vi "Logging Message Loop.vi"(8 "error in (no error)":errorcluster, 10 "Data Queue":refnum<queue>, 11 "Message Queues":T1) -> (0 "error out":errorcluster)   [LabVIEW 2013, in "Logging.lvlib"]
doc: "The message loop subVI to handle messages pertaining to logging data."
uses:
  Logging.lvlib
  support/Message Queue/All Message Queues.ctl
  support/Message Queue/Message Cluster.ctl
  Logging Configuration.ctl
  Logging State.ctl
  controls/UI Data.ctl
  <vilib>/Utility/error.llb/DialogType.ctl
  support/Message Queue/Enqueue Message (Single).vi
  <vilib>/ErrorRing/Error Ring.xnode
  support/Message Queue/Message Queue.lvlib
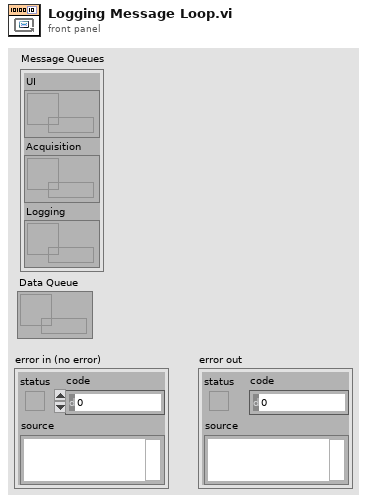
[diagram p1: front panel]
types:
  T1 = typedef "Message Queue.lvlib/All Message Queues.ctl" = cluster{"UI":refnum<queue>, "Acquisition":refnum<queue>, "Logging":refnum<queue>}
  T2 = cluster{"Macro:Initialize":string, "Macro:Exit":string, "Core":cluster{"Current VI Reference":refnum<vi>, "Close Panel on Exit?":bool}}
  T3 = typedef "UI Data.ctl" = cluster{"Start Ref":refnum<vi>, "Stop Ref":refnum<vi>, "Settings Ref":refnum<vi>, "Exit Ref":refnum<vi>, "Status Ref":refnum<vi>, "Data Ref":refnum<vi>}
  T4 = typedef "Logging.lvlib/Logging State.ctl" = enum16{"Idle", "Logging"}
  T5 = typedef "Logging.lvlib/Logging Configuration.ctl" = cluster{"Log File Base Path":path, "TDMS File Reference":refnum<k34>}
  T6 = enum32{"invalid app kind", "Development System", "Run Time System", "Student Edition", "Embedded LabVIEW", "Evaluation", "Custom"}
  T7 = typedef "Message Queue.lvlib/Message Cluster.ctl" = cluster{"Message":string, "Message Data":variant}
  T8 = enum32{"Invalid", "Standard", "Closed", "Hidden", "Minimized", "Maximized"}
  T9 = enum16{"open", "open or create", "create or replace", "create", "open (read-only)"}
  T10 = typedef "DialogType.ctl" = u16
  T11 = cluster{"element":T7, "error constant":errorcluster}
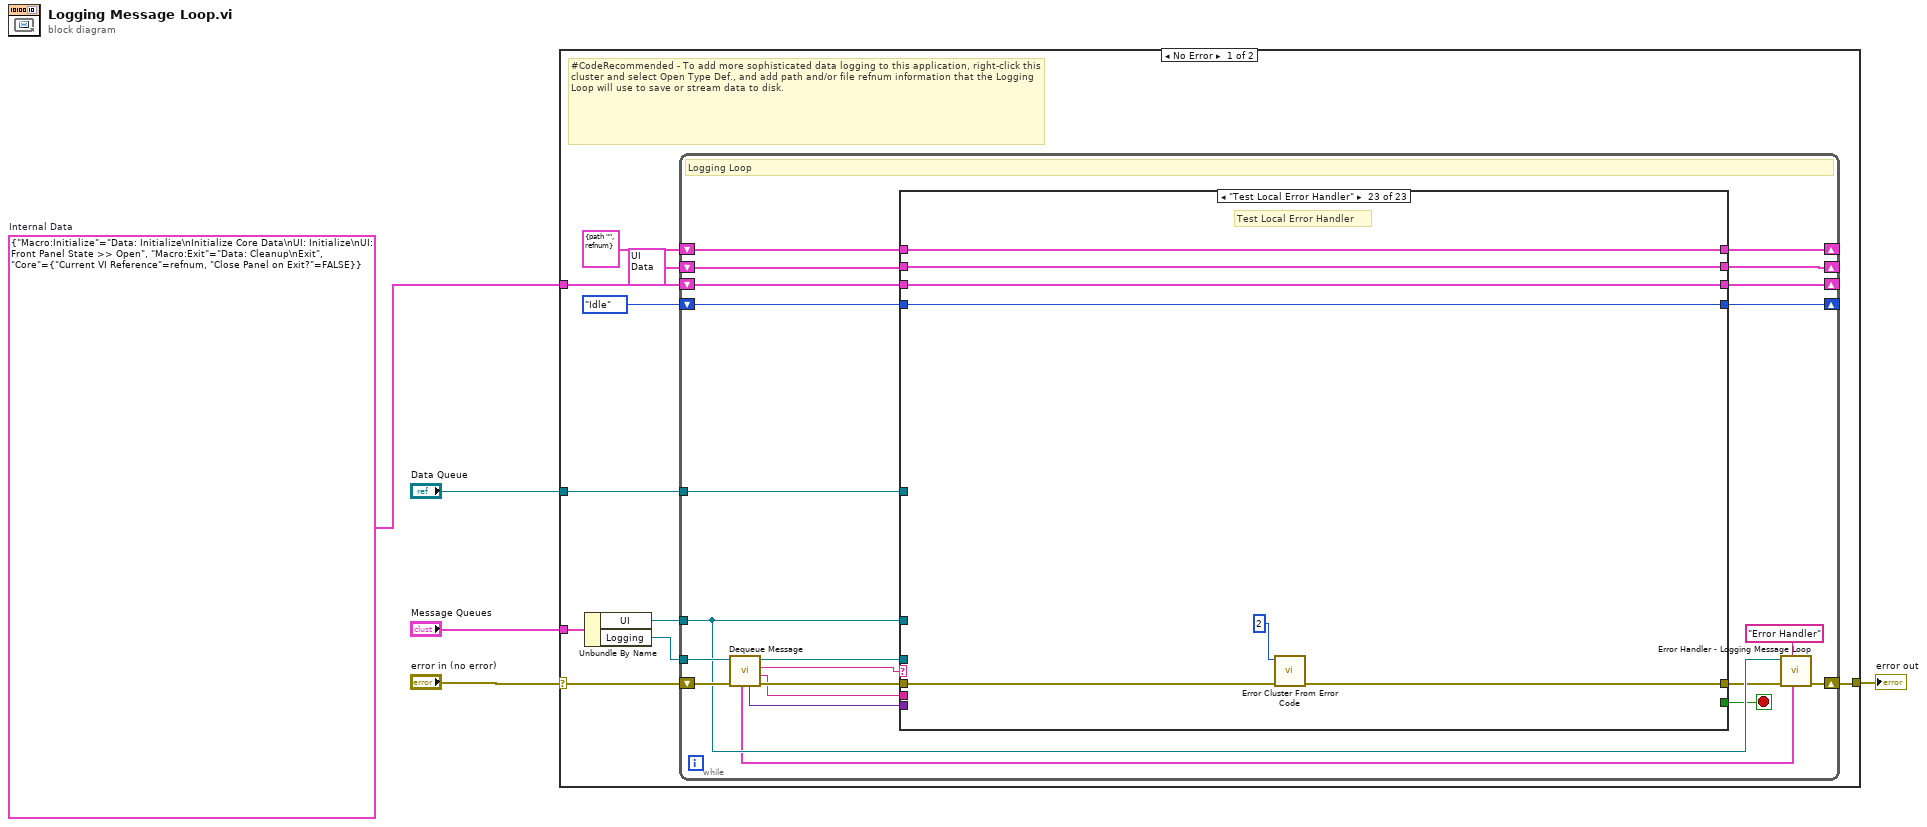
[diagram p0: block diagram]
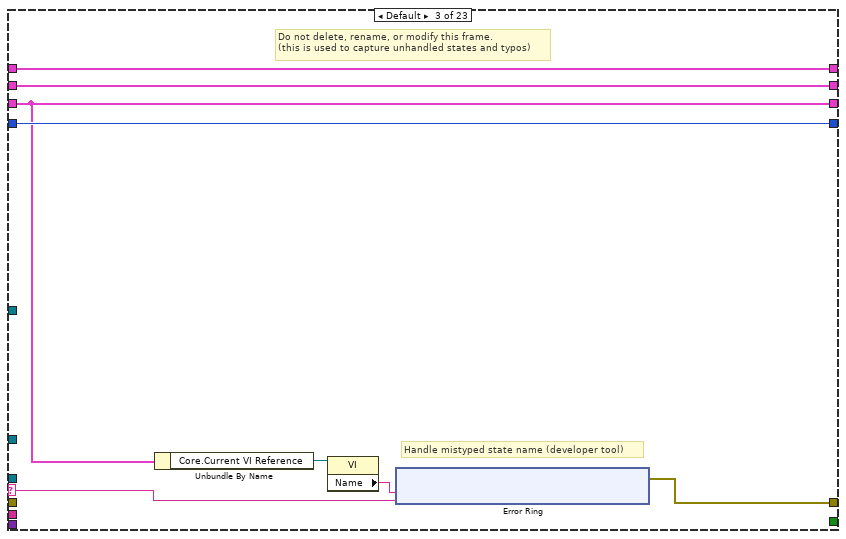
[diagram p4: hidden frame]
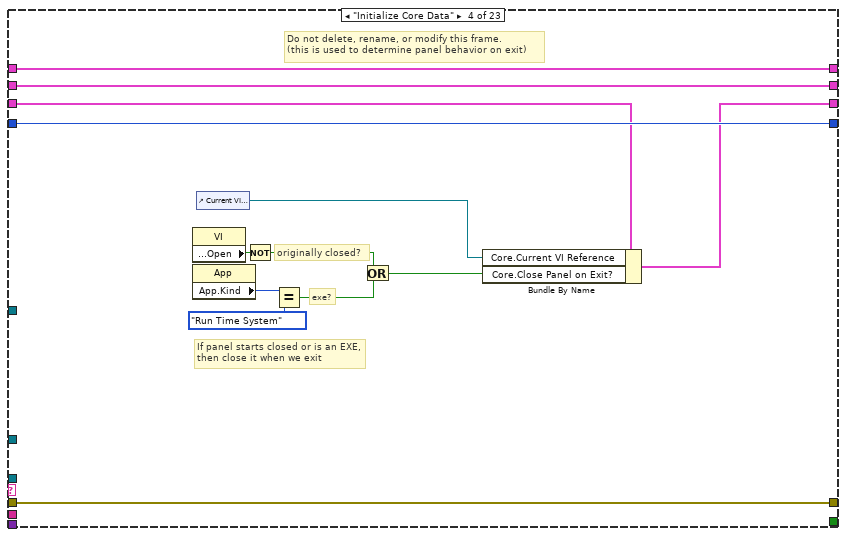
[diagram p5: hidden frame]
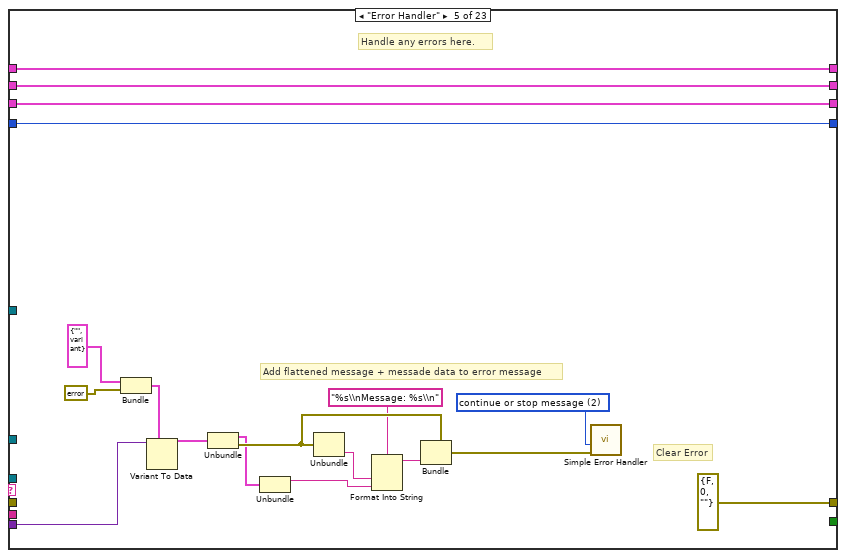
[diagram p6: hidden frame]
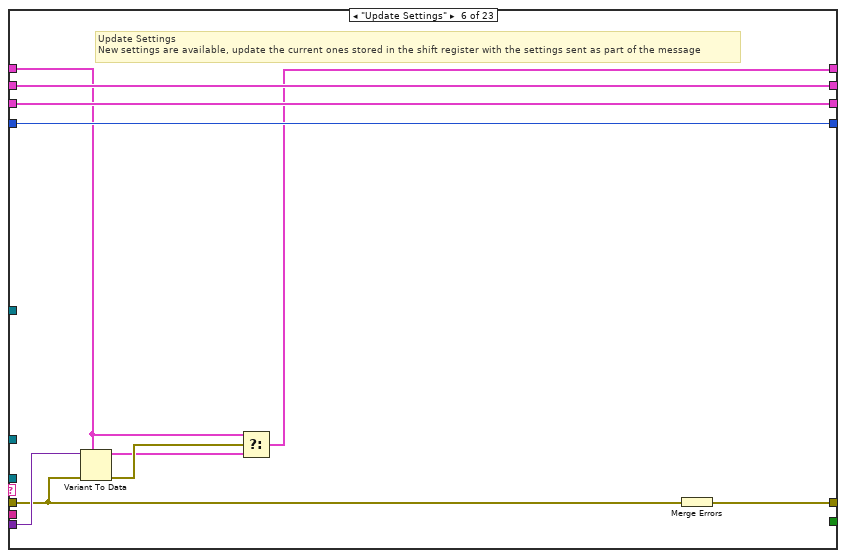
[diagram p7: hidden frame]
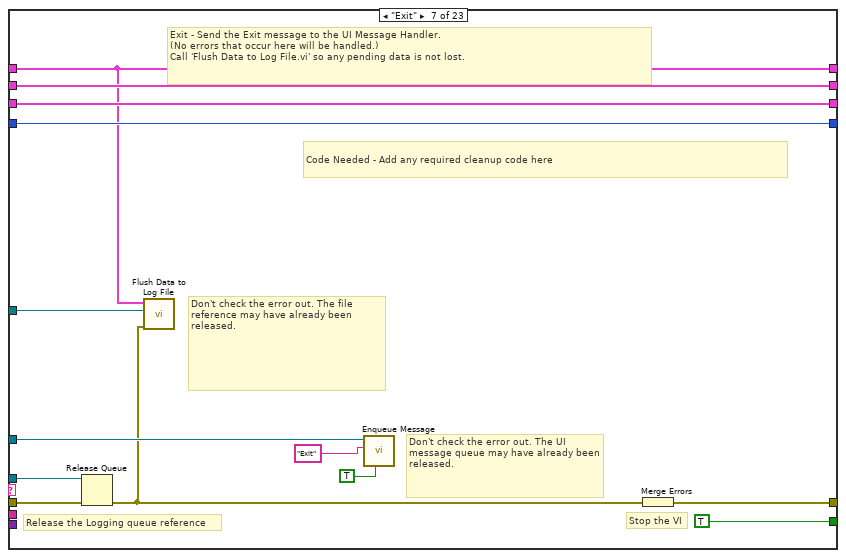
[diagram p8: hidden frame]
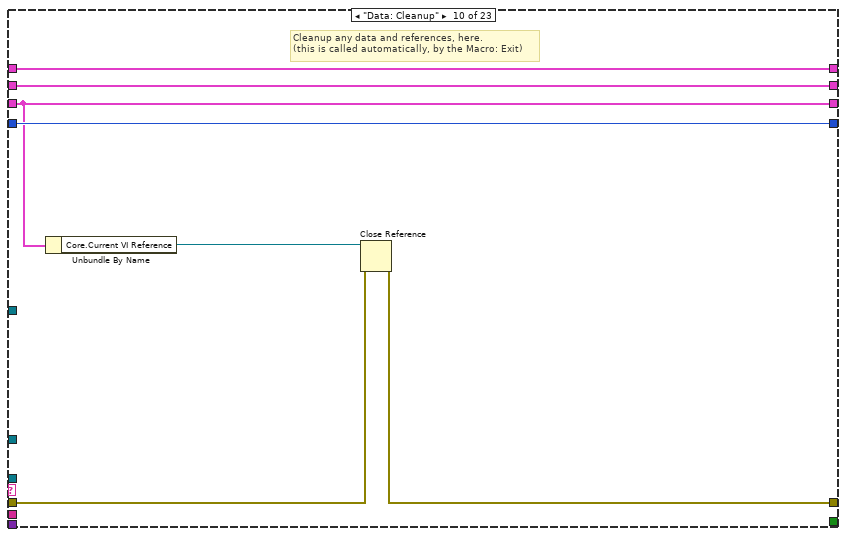
[diagram p11: hidden frame]
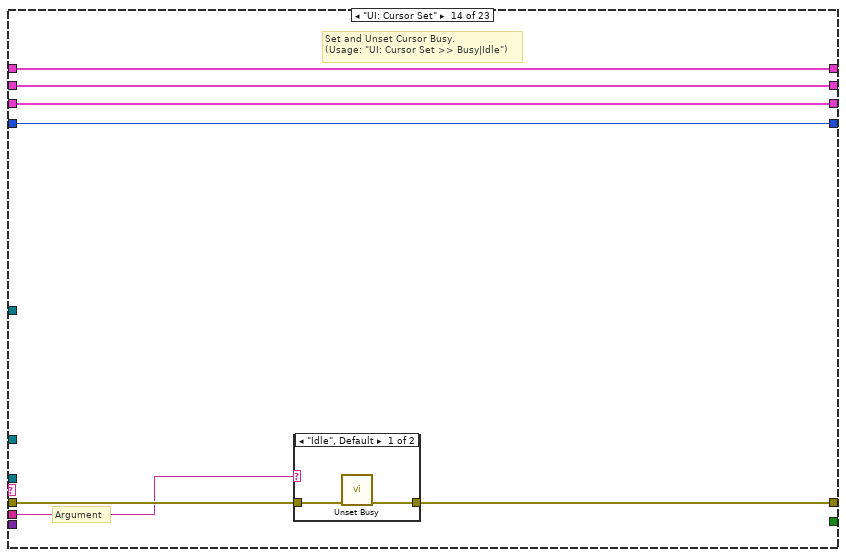
[diagram p15: hidden frame]
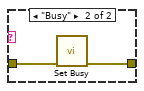
[diagram p16: hidden frame]
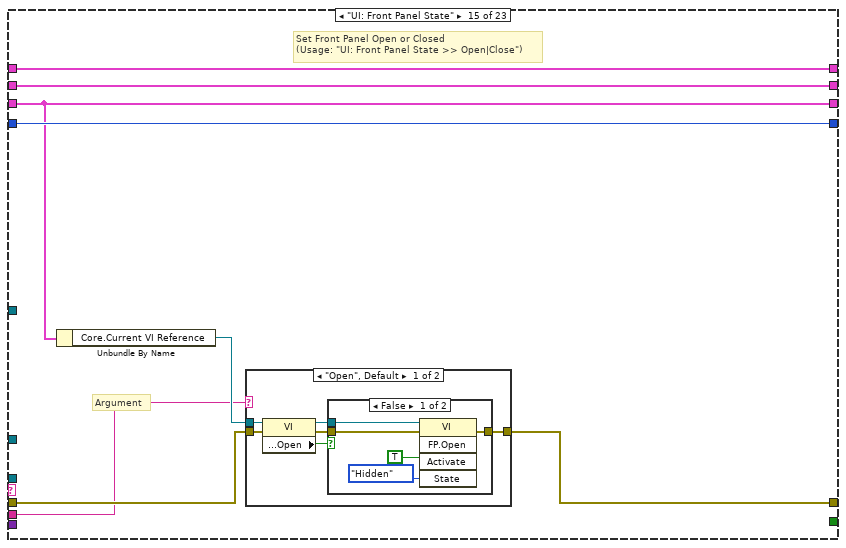
[diagram p17: hidden frame]
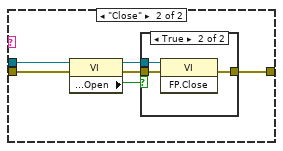
[diagram p19: hidden frame]
diagram:
  w1 = T2 {"Macro:Initialize"="Data: Initialize\nInitialize Core Data\nUI: Initialize\nUI: Front Panel State >> Open", "Macro:Exit"="Data: Cleanup\nExit", "Core"={"Current VI Reference"=refnum, "Close Panel on Exit?"=FALSE}}  # Internal Data
  n1 = case shown="No Error" "error in (no error)" {
    selector: "error in (no error)" -> [w11 w307]
    tunnel: "Message Queues" -> [w15 _]
    tunnel: [w13 w307] -> w4
    tunnel: "Data Queue" -> [w10 _]
    tunnel: w1 -> [w7 _]
    frame No Error {
      # "#CodeRecommended - To add more sophisticated data logging to this application, right-click this cluster and select Open Type Def., and add path and/or file refnum information that the Logging Loop will use to save or stream data to disk."
      n2 = Unbundle By Name(w15) -> ("UI"=w9:refnum<queue>, "Logging"=w14:refnum<queue>)
      n3 = while {
        tunnel: w14 -> [w36]
        shift-right: [w25] -> _
        shift-left: T5 {"Log File Base Path"=path "", "TDMS File Reference"=refnum} ("Logging Configuration") -> [w26]
        shift-right: [w35] -> w13
        shift-left: w11 -> [w37]
        tunnel: w9 -> [w33]
        tunnel: w10 -> [w20]
        shift-right: [w23] -> _
        shift-left: Logging_State."Idle" ("State") -> [w24]
        shift-right: [w19] -> _
        shift-left: T3 {"Start Ref"=refnum, "Stop Ref"=refnum, "Settings Ref"=refnum, "Exit Ref"=refnum, "Status Ref"=refnum, "Data Ref"=refnum} ("Measurement UI Controls") -> [w21]
        shift-right: [w18] -> _
        shift-left: w7 -> [w22]
        stop <- w28 stop-if-true
        # "Logging Loop"
        n4 = call "Dequeue Message.vi"("error in (no error)"=w37, "Message Queue"=w36) -> ("error out"=w34:errorcluster, "Argument"=w30:string, "Message"=w31:string, "dup Message Queue"=w32:refnum<queue>, "Message Data"=w29:variant, "element"=w16:T7)  [unwired: 4 in]
        n5 = case shown="\"Test Local Error Handler\"" w31 {
          selector: w31 -> [_ _ w50 _ _ _ _ _ _ _ _ _ _ _ _ _ _ _ _ _ w261 _ _]
          tunnel: w21 -> [w41 w45 w54 w68 w94 w104 w116 w120 w127 w130 w137 w142 w147 w152 w163 w193 w202 w216 w222 w229 w264 w288 w305]
          tunnel: w30 -> [_ _ _ _ _ _ _ _ _ _ _ _ _ w153 w164 _ _ _ _ _ _ _ _]
          tunnel: w26 -> [w40 w46 w55 w66 w92 w98 w106 w121 w123 w131 w138 w144 w149 w156 w166 w194 w203 w214 w223 w230 w259 w279 w304]
          tunnel: [w42 w47 w48 w76 errorcluster {"status"=FALSE, "code"=0, "source"=""} ("error out") w96 w108 w122 w124 w132 w139 w143 w148 w154 w167 w195 w198 w204 w224 w227 w262 w284 w300] -> w27
          tunnel: w34 -> [w42 w47 _ w76 _ w95 w113 w122 w124 w133 w139 w143 w148 w155 w168 w195 w200 w213 w224 w226 w260 w283 w301]
          tunnel: [w41 w45 w54 w68 w94 w104 w116 w120 w127 w130 w137 w142 w147 w152 w163 w193 w202 w216 w222 w229 w264 w288 w305] -> w19
          tunnel: [_ _ _ _ _ _ TRUE _ _ _ _ _ _ _ _ _ _ _ _ _ _ _ _] -> w28
          tunnel: [w40 w46 w55 w66 w92 w97 w106 w121 w123 w131 w138 w144 w149 w156 w166 w194 w203 w214 w223 w231 w259 w278 w304] -> w25
          tunnel: [w39 w44 w53 w67 w93 w103 w115 w119 w126 w129 w136 w141 w146 w151 w162 w192 w201 w215 w221 w228 w263 w286 w303] -> w23
          tunnel: w24 -> [w39 w44 w53 w67 w93 w103 w115 w119 w126 w129 w136 w141 w146 w151 w162 w192 w201 w215 w221 w232 w265 w287 w303]
          tunnel: w29 -> [_ _ _ _ w77 w101 _ _ _ _ _ _ _ _ _ _ _ _ _ _ _ _ _]
          tunnel: w22 -> [w38 w43 w49 w65 w91 w102 w114 w118 w125 w128 w135 w140 w145 w150 w161 w191 w196 w207 w220 w233 w266 w289 w306]
          tunnel: [w38 w43 w49 w64 w91 w102 w114 w118 w125 w128 w135 w140 w145 w150 w161 w191 w196 w207 w220 w233 w266 w289 w306] -> w18
          tunnel: w32 -> [_ _ _ _ _ _ w112 _ _ _ _ _ _ _ _ _ w199 w212 _ w225 w257 _ _]
          tunnel: w33 -> [_ _ _ _ _ _ w111 _ _ _ _ _ _ _ _ _ _ _ _ _ _ w281 _]
          tunnel: w20 -> [_ _ _ _ _ _ w107 _ _ _ _ _ _ _ _ _ _ _ _ _ w258 w282 _]
          frame "", "Idle" {
            # "Executes when the state queue is empty\nAlso commented out messages"
          }
          frame "---------- Core ----------" {
            # "Do not put any code in this frame.\n(it is a separator no-op)"
          }
          frame Default {
            # "Handle mistyped state name (developer tool)"
            # "Do not delete, rename, or modify this frame.\n(this is used to capture unhandled states and typos)"
            n6 = Unbundle By Name(w49) -> ("Core.Current VI Reference"=w51:refnum<vi>)
            n7 = property class="VI"(reference=w51) -> ("Name"=w52:string)  [unwired: 1 in, 2 out]
            n8 = xnode "Error Ring"("parameter 0"=w52, "parameter 1"=w50) -> ("error out"=w48:errorcluster)
          }
          frame "Initialize Core Data" {
            # "Do not delete, rename, or modify this frame.\n(this is used to determine panel behavior on exit)"
            # "originally closed?"
            # "exe?"
            # "If panel starts closed or is an EXE, then close it when we exit"
            n9 = property class="VI"() -> ("Front Panel.Open"=w75:bool)  [unwired: 2 in, 2 out]
            n10 = property class="App"() -> ("App.Kind"=w74:T6)  [unwired: 2 in, 2 out]
            n11 = control-ref of="Current VI Reference"() -> (w69:refnum<vi>)
            n12 = Not(x=w75) -> (.not. x?=w72:bool)
            n13 = Equal?(x=w74, y=T6."Run Time System" ("Application:Kind")) -> (x = y?=w71:bool)
            n14 = Or(x=w72, y=w71) -> (x .or. y?=w70:bool)
            n15 = Bundle By Name(cluster=w65, "Core.Current VI Reference"=w69, "Core.Close Panel on Exit?"=w70) -> (w64:T2)
          }
          frame "Error Handler" {
            w89 = T10 2 items=["no dialog", "OK message", "continue or stop message", "OK message + warnings", "continue/stop + warnings"] ("type of dialog (OK msg:1)")
            # "Add flattened message + messade data to error message"
            # "Clear Error"
            # "Handle any errors here."
            n16 = Bundle("element"=T7 {"Message"="", "Message Data"=variant}, "error constant"=errorcluster {"status"=FALSE, "code"=0, "source"=""}) -> (w86:T11)  [unwired: 1 in]
            n17 = Variant To Data(type=w86, Variant=w77) -> (data=w85:T11)  [unwired: 1 in, 1 out]
            n18 = Unbundle(w85) -> ("element"=w82:T7, "error constant"=w84:errorcluster)
            n19 = Unbundle(w82) -> ("Message"=w80:string)  [unwired: 1 out]
            n20 = Unbundle(w84) -> ("source"=w79:string)  [unwired: 2 out]
            n21 = Format Into String(format string="%s\\nMessage: %s\\n", w79, w80) -> (resulting string=w81:string)  [unwired: 2 in, 1 out]
            n22 = Bundle(cluster=w84, "source"=w81) -> (w83:errorcluster)  [unwired: 2 in]
            n23 = call <vilib>:"Simple Error Handler.vi"("type of dialog (OK msg:1)"=w89, "error in (no error)"=w83) -> ()  [unwired: 3 in, 5 out]
          }
          frame "Update Settings" {
            # "Update Settings\nNew settings are available, update the current ones stored in the shift register with the settings sent as part of the message"
            n24 = Variant To Data(error in=w95, type=w98, Variant=w101) -> (data=w99:T5, error out=w100:errorcluster)
            n25 = Select(t=w98, s=w100, f=w99) -> (s? t:f=w97:T5)
            n26 = Merge Errors(w95) -> (w96:errorcluster)
          }
          frame "Exit" {
            # "Stop the VI"
            # "Don't check the error out. The file reference may have already been released."
            # "Code Needed - Add any required cleanup code here"
            # "Exit - Send the Exit message to the UI Message Handler.\n(No errors that occur here will be handled.)\nCall 'Flush Data to Log File.vi' so any pending data is not lost."
            # "Don't check the error out. The UI message queue may have already been released."
            # "Release the Logging queue reference"
            n27 = Release Queue(queue=w112, error in (no error)=w113) -> (error out=w105:errorcluster)  [unwired: 1 in, 2 out]
            n28 = call "Flush Data to Log File.vi"("error in (no error)"=w105, "Data Queue"=w107, "Logging Configuration"=w106) -> ()  [unwired: 8 in, 1 out]
            n29 = call-poly "Enqueue Message.vi"("Priority Message? (F)"=TRUE, "Message"="Exit", "Message Queue"=w111) -> ()  [unwired: 7 in, 2 out]
            n30 = Merge Errors(w105) -> (w108:errorcluster)
          }
          frame "---------- Data ----------" {
            # "Do not put any code in this frame.\n(It is a separator no-op. You can make a copy of this frame to create a new Data frame)"
          }
          frame "Data: Initialize" {
            # "nothing right now"
            # "Initialize the shift-register data, here.\n(data names are defined by what you wire into the bundle function)"
          }
          frame "Data: Cleanup" {
            # "Cleanup any data and references, here.\n(this is called automatically, by the Macro: Exit)"
            n31 = Unbundle By Name(w128) -> ("Core.Current VI Reference"=w134:refnum<vi>)
            n32 = Close Reference(reference=w134, error in (no error)=w133) -> (error out=w132:errorcluster)
          }
          frame "---------- UI ----------" {
            # "Do not put any code in this frame.\n(It is a separator no-op. You can make a copy of this frame to create a new UI frame)"
          }
          frame "UI: Initialize" {
            # "Initialize the User Interface, here.\n(this is called automatically, by the Macro: Init)"
          }
          frame "UI: Initialize UI Refs" {
            # "Package and Init UI Refs as Required"
          }
          frame "UI: Cursor Set" {
            # "Argument"
            # "Set and Unset Cursor Busy.\n(Usage: \"UI: Cursor Set >> Busy|Idle\")"
            n33 = case shown="\"Idle\", Default" w153 {
              tunnel: w155 -> [w158 w160]
              tunnel: [w157 w159] -> w154
              frame "Idle", Default {
                n34 = call <vilib>:"Unset Busy.vi"("error in (no error)"=w158) -> ("error out"=w157:errorcluster)  [unwired: 10 in]
              }
              frame "Busy" {
                n35 = call <vilib>:"Set Busy.vi"("error in (no error)"=w160) -> ("error out"=w159:errorcluster)  [unwired: 9 in, 1 out]
              }
            }
          }
          frame "UI: Front Panel State" {
            # "Argument"
            # "Set Front Panel Open or Closed\n(Usage: \"UI: Front Panel State >> Open|Close\")"
            n36 = Unbundle By Name(w161) -> ("Core.Current VI Reference"=w165:refnum<vi>)
            n37 = case shown="\"Open\", Default" w164 {
              tunnel: w168 -> [w172 w185]
              tunnel: [w174 w186] -> w167
              tunnel: w165 -> [w173 w183]
              frame "Open", Default {
                n38 = property class="VI"(reference=w173, error in=w172) -> (reference out=w170:refnum<vi>, error out=w171:errorcluster, "Front Panel.Open"=w169:bool)
                n39 = case shown="False" w169 {
                  tunnel: [w177 w180] -> w174
                  tunnel: w171 -> [w176 w180]
                  tunnel: w170 -> [w175 _]
                  frame False {
                    n40 = invoke class="VI" method="FP.Open"(reference=w175, error in=w176, "Activate"=TRUE, "State"=T8."Hidden") -> (error out=w177:errorcluster)  [unwired: 1 in, 4 out]
                  }
                  frame True {
                  }
                }
              }
              frame "Close" {
                n41 = property class="VI"(reference=w183, error in=w185) -> (reference out=w182:refnum<vi>, error out=w184:errorcluster, "Front Panel.Open"=w181:bool)
                n42 = case shown="True" w181 {
                  tunnel: [w187 w190] -> w186
                  tunnel: w184 -> [w187 w189]
                  tunnel: w182 -> [_ w188]
                  frame False {
                  }
                  frame True {
                    n43 = invoke class="VI" method="FP.Close"(reference=w188, error in=w189) -> (error out=w190:errorcluster)  [unwired: 1 in, 2 out]
                  }
                }
              }
            }
          }
          frame "---------- Macro ----------" {
            # "Do not put any code in this frame.\n(It is a separator no-op. You can make a copy of this frame to create a new Macro frame)"
          }
          frame "Macro: Initialize" {
            # "Initialization Macro\n(This is called once, when the VI starts)"
            n44 = Unbundle By Name(w196) -> ("Macro:Initialize"=w197:string)
            n45 = call-poly "Enqueue Message.vi"("error in (no error)"=w200, "Message"=w197, "Message Queue"=w199) -> ("error out"=w198:errorcluster)  [unwired: 7 in, 1 out]
          }
          frame "Macro: Exit" {
            # "Exit Macro\n(This is called once, when the VI exits)"
            n46 = Unbundle By Name(w207) -> ("Core.Close Panel on Exit?"=w219:bool)
            n47 = Unbundle By Name(w207) -> ("Macro:Exit"=w206:string)
            n48 = Select(t="UI: Front Panel State >> Close", s=w219, f="") -> (s? t:f=w211:string)
            n49 = call-poly "Enqueue Message.vi"("Priority Message? (F)"=TRUE, "error in (no error)"=w213, "Message"=w211, "Message Queue"=w212) -> ("error out"=w208:errorcluster, "dup Message Queue"=w209:refnum<queue>)  [unwired: 6 in]
            n50 = call-poly "Enqueue Message.vi"("Priority Message? (F)"=FALSE, "error in (no error)"=w208, "Message"=w206, "Message Queue"=w209) -> ("error out"=w204:errorcluster)  [unwired: 6 in, 1 out]
          }
          frame "---------- Log ----------" {
            # "Logging Section"
          }
          frame "Start" {
            # "Start - Send the \"Log\" message to start logging. \nGenerate a unique, timestamped TDMS file name based on the Log File Base Path value."
            n51 = case shown="\"Idle\"" w232 {
              selector: w232 -> [w236 _]
              tunnel: [w234 w242] -> w227
              tunnel: [w236 Logging_State."Logging" ("State")] -> w228
              tunnel: w230 -> [w235 w240]
              tunnel: [w235 w241] -> w231
              tunnel: w226 -> [w234 w238]
              tunnel: w225 -> [_ w237]
              frame "Logging" {
                # "The system is already logging. Ignore the \"Start\" message."
              }
              frame "Idle" {
                # "If the system is idle, start logging."
                n52 = Unbundle By Name(w240) -> ("Log File Base Path"=w239:path)
                n53 = Strip Path(path=w239) -> (stripped path=w253:path)  [unwired: 1 out]
                n54 = call <vilib>:"Get File Extension.vi"("file"=w239) -> ("filename without extension"=w254:string, "lowercase file extension"=w250:string)  [unwired: 7 in, 2 out]
                n55 = Format Date/Time String(time format string (%c)="%Y_%m_%d_%H_%M_%S") -> (date/time string=w251:string)  [unwired: 2 in]
                n56 = Format Into String(format string="_%s.%s", initial string=w254, w251, w250) -> (resulting string=w249:string)  [unwired: 1 in, 1 out]
                n57 = Build Path(base path=w253, name or relative path=w249) -> (appended path=w248:path)
                n58 = call-poly "Enqueue Message.vi"("error in (no error)"=w238, "Message"="Log", "Message Queue"=w237) -> ("error out"=w246:errorcluster)  [unwired: 7 in, 1 out]
                n59 = TDMS Open(8:w238, 10:T9."create or replace" ("operation (0:open)"), 11:w248) -> (0:w247:errorcluster, 3:w244:refnum<k34>)  [unwired: 4 in]
                n60 = Merge Errors(w247, w246) -> (w242:errorcluster)
                n61 = Bundle By Name(cluster=w240, "TDMS File Reference"=w244) -> (w241:T5)
              }
            }
          }
          frame "Log" {
            # "Log - Log data to disk.\nSince this is a continuous acquisition, this message will always message itself to run again."
            n62 = case shown="\"Logging\"" w265 {
              selector: w265 -> [w268 w274]
              tunnel: [w267 w277] -> w262
              tunnel: [w268 w274] -> w263
              tunnel: w261 -> [_ w273]
              tunnel: w260 -> [w267 w270]
              tunnel: w259 -> [_ w272]
              tunnel: w258 -> [_ w271]
              tunnel: w257 -> [_ w269]
              frame "Idle" {
                # "Ignore \"Log\" messages when the logging is idle."
              }
              frame "Logging" {
                # "Log more data while in the \"Logging\" state."
                n63 = call "Log Data.vi"("error in (no error)"=w270, "Data Queue"=w271, "Logging Configuration"=w272) -> ("error out"=w275:errorcluster)  [unwired: 8 in]
                n64 = call-poly "Enqueue Message.vi"("error in (no error)"=w270, "Message"=w273, "Message Queue"=w269) -> ("error out"=w276:errorcluster)  [unwired: 7 in, 1 out]
                n65 = Merge Errors(w275, w276) -> (w277:errorcluster)
              }
            }
          }
          frame "Stop" {
            # "Log - Log data to disk.\nSince this is a continuous acquisition, this message will always message itself to run again."
            n66 = case shown="\"Logging\"" w287 {
              selector: w287 -> [w291 _]
              tunnel: [w290 w297] -> w285
              tunnel: [w291 Logging_State."Idle" ("State")] -> w286
              tunnel: w283 -> [w290 w295]
              tunnel: w282 -> [_ w294]
              tunnel: w279 -> [_ w293]
              tunnel: w281 -> [_ w292]
              frame "Idle" {
                # "The system is already idle. Ignore the \"Stop\" message."
              }
              frame "Logging" {
                # "If the system is logging, stop logging."
                n67 = call "Flush Data to Log File.vi"("error in (no error)"=w295, "Data Queue"=w294, "Logging Configuration"=w293) -> ("error out"=w299:errorcluster)  [unwired: 8 in]
                n68 = call-poly "Enqueue Message.vi"("error in (no error)"=w299, "Message"="Logging Stopped", "Message Queue"=w292) -> ("error out"=w297:errorcluster)  [unwired: 7 in, 1 out]
              }
            }
            n69 = Merge Errors(w285) -> (w284:errorcluster)
            n70 = Bundle By Name(cluster=w279, "TDMS File Reference"=refnum<k34> refnum) -> (w278:T5)
          }
          frame "Test Local Error Handler" {
            # "Test Local Error Handler"
            n71 = call <vilib>:"Error Cluster From Error Code.vi"("error in (no error)"=w301, "error code (0)"=2) -> ("error out"=w300:errorcluster)  [unwired: 7 in]
          }
        }
        n72 = call "Error Handler - Logging Message Loop.vi"("element"=w16, "Error Handler Message"="Error Handler" ("Message"), "error in (no error)"=w27, "Message Queue"=w33) -> ("dup error in"=w35:errorcluster)  [unwired: 6 in, 1 out]
      }
    }
    frame Error {
    }
  }
  "error out" <- w4
